vi "GOMDBTS2048 get CQS.vi"(0 "handle":i32, 7 "error in (no error)":errorcluster) -> (10 "Q15":dbl, 11 "function return":i32, 12 "Q13":dbl, 13 "Q14":dbl, 14 "Q11":dbl, 15 "Q12":dbl, 16 "Q9":dbl, 17 "Q10":dbl, 18 "Q7":dbl, 19 "Q8":dbl, 20 "Qa":dbl, 21 "Q1":dbl, 22 "Q2":dbl, 23 "Q3":dbl, 24 "Q4":dbl, 25 "Q5":dbl, 26 "Q6":dbl, 27 "error out":errorcluster)   [LabVIEW 2015, in "GOMDBTS2048.lvlib"]
doc: "GOBTS2048DLL int __stdcall GOMDBTS2048_getCRI(int handle, double* Ra, double* R1, double* R2, double* R3, double* R4, double* R5, double* R6,\n double* R7, double* R8, double* R9, double* R10, double* R11, double* R12, double* R13, double* R14, double* R15);"
uses:
  GOMDBTS2048.lvlib
  runtime/GOMDBTS2048.dll
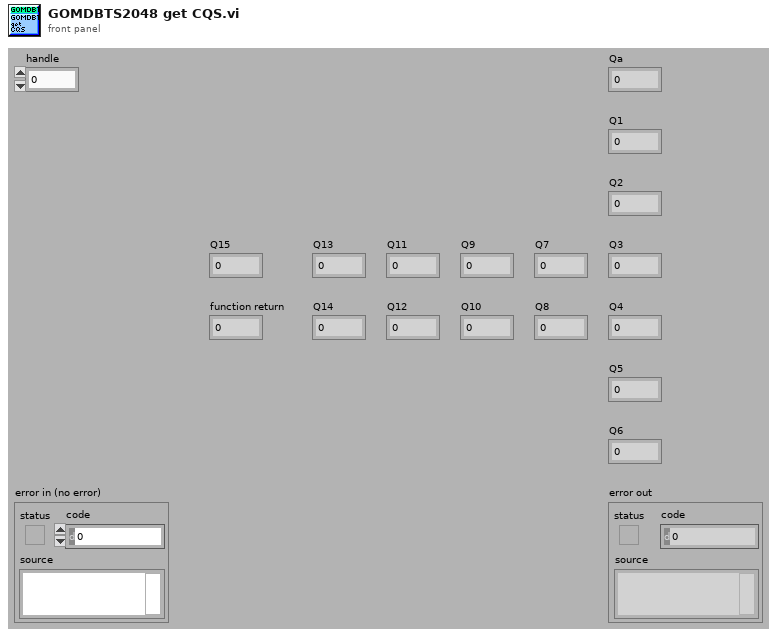
[diagram p1: front panel]
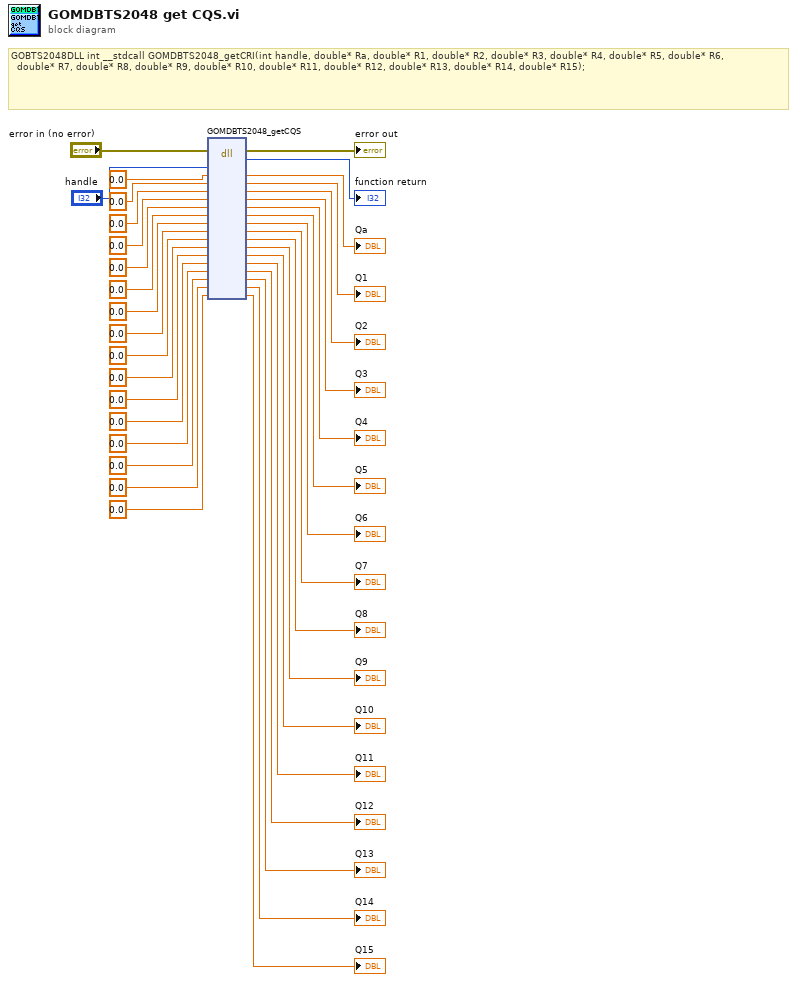
[diagram p0: block diagram]
diagram:
  # "GOBTS2048DLL int __stdcall GOMDBTS2048_getCRI(int handle, double* Ra, double* R1, double* R2, double* R3, double* R4, double* R5, double* R6,\n\t\tdouble* R7, double* R8, double* R9, double* R10, double* R11, double* R12, double* R13, double* R14, double* R15);"
  n1 = dll-call lib="C:/Users/rkoch/Documents/GO_Library/runtime/GOMDBTS2048.*" fn="GOMDBTS2048_getCQS"(error in="error in (no error)", "handle"="handle", "Qa"=0.0 ("Ra"), "Q1"=0.0 ("R1"), "Q2"=0.0 ("R2"), "Q3"=0.0 ("R3"), "Q4"=0.0 ("R4"), "Q5"=0.0 ("R5"), "Q6"=0.0 ("R6"), "Q7"=0.0 ("R7"), "Q8"=0.0 ("R8"), "Q9"=0.0 ("R9"), "Q10"=0.0 ("R10"), "Q11"=0.0 ("R11"), "Q12"=0.0 ("R12"), "Q13"=0.0 ("R13"), "Q14"=0.0 ("R14"), "Q15"=0.0 ("R15")) -> (error out=→"error out":errorcluster, "return type"=→"function return":i32, "Qa"=→"Qa":dbl, "Q1"=→"Q1":dbl, "Q2"=→"Q2":dbl, "Q3"=→"Q3":dbl, "Q4"=→"Q4":dbl, "Q5"=→"Q5":dbl, "Q6"=→"Q6":dbl, "Q7"=→"Q7":dbl, "Q8"=→"Q8":dbl, "Q9"=→"Q9":dbl, "Q10"=→"Q10":dbl, "Q11"=→"Q11":dbl, "Q12"=→"Q12":dbl, "Q13"=→"Q13":dbl, "Q14"=→"Q14":dbl, "Q15"=→"Q15":dbl)  [unwired: 3 in, 1 out]
